vi "Colour selector.vi"(4 "Colour":string(combo), 11 "Error in":errorcluster) -> (15 "Error out":errorcluster)   [LabVIEW 2020]
uses:
  <vilib>/Utility/miscctls.llb/LVPositionTypeDef.ctl
panel:
  in  "Next":bool
  # "Catch and select the colour"
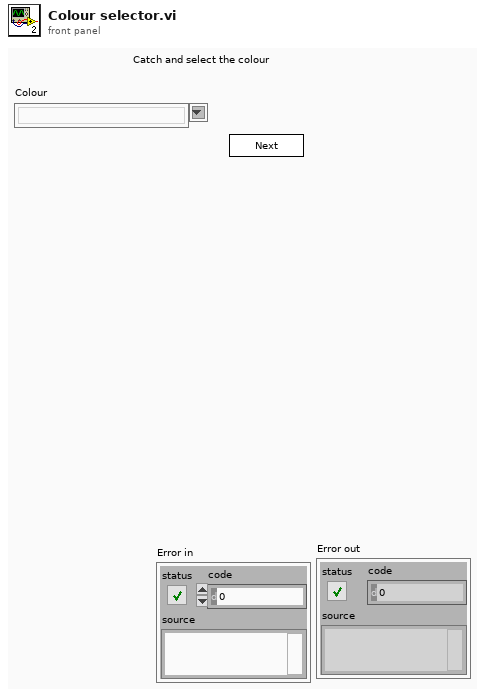
[diagram p1: front panel]
types:
  T1 = typedef "LVPositionTypeDef.ctl" = cluster{"Left":i32, "Top":i32}
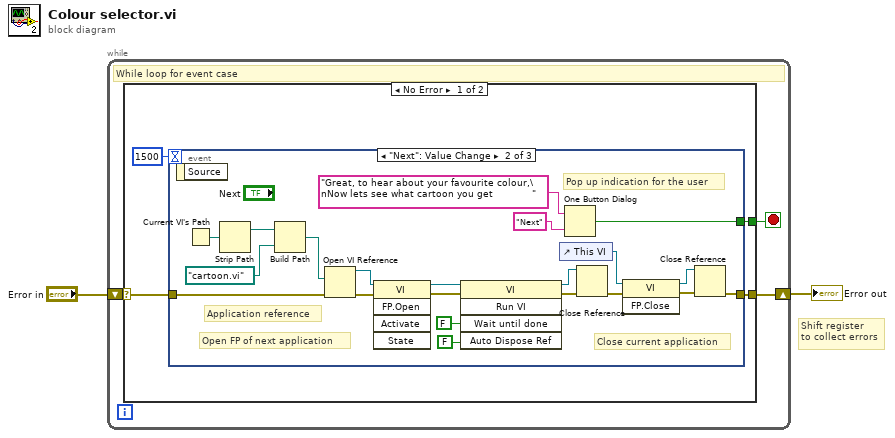
[diagram p0: block diagram]
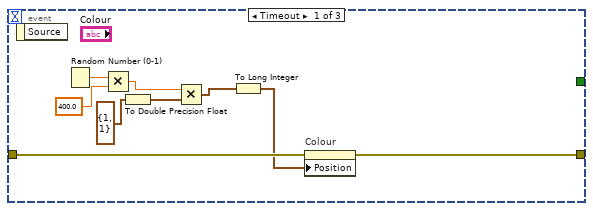
[diagram p2: hidden frame]
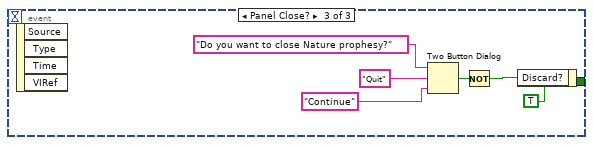
[diagram p3: hidden frame]
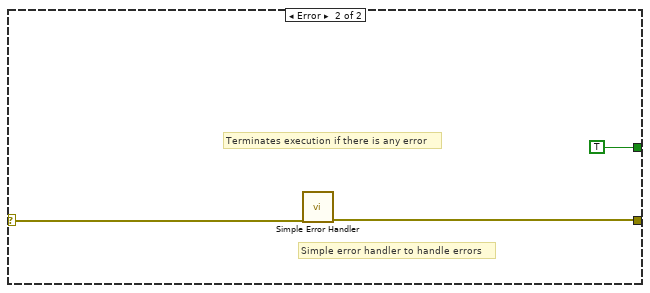
[diagram p4: hidden frame]
diagram:
  # "Shift register \nto collect errors"
  n1 = while {
    shift-right: [w4] -> w1
    shift-left: "Error in" -> [w5]
    stop <- w3 stop-if-true
    # "While loop for event case"
    n2 = case shown="No Error" w5 {
      selector: w5 -> [w9 w48]
      tunnel: [w8 w47] -> w4
      tunnel: [w7 TRUE] -> w3
      frame No Error {
        n3 = event shown="[1] \"Next\": Value Change" {
          selector: _ -> [_ _ _]
          dyn-events: _ -> [_ _ _]
          timeout: 1500 -> [_ _ _]
          tunnel: [w17 w26 _] -> w8
          tunnel: w9 -> [w18 w31 _]
          tunnel: [_ w25 TRUE] -> w7
          event Timeout {
            n4 = event-data() -> ()  [unwired: 1 in, 1 out]
            n5 = Random Number (0-1)() -> (number: 0 to 1=w16:dbl)
            n6 = Multiply(x=w16, y=400.0) -> (x*y=w14:dbl)
            n7 = To Double Precision Float(number=T1 {"Left"=1, "Top"=1} ("Position")) -> (double precision float=w13:cluster{"Left":dbl, "Top":dbl})
            n8 = Multiply(x=w14, y=w13) -> (x*y=w11:cluster{"Left":dbl, "Top":dbl})
            n9 = To Long Integer(number=w11) -> (32bit integer=w10:cluster{"Left":i32, "Top":i32})
            n10 = property on="Colour" class="CmbBox"(error in=w18, "Position"=w10) -> (error out=w17:errorcluster)  [unwired: 1 in, 1 out]
          }
          event "Next": Value Change {
            # "Pop up indication for the user"
            # "Close current application"
            # "Application reference"
            # "Open FP of next application"
            n11 = event-data() -> ()  [unwired: 1 in, 1 out]
            n12 = Current VI's Path() -> (path=w36:path)
            n13 = Strip Path(path=w36) -> (stripped path=w35:path)  [unwired: 1 out]
            n14 = Build Path(base path=w35, name or relative path=path "cartoon.vi") -> (appended path=w34:path)
            n15 = Open VI Reference(vi path=w34, error in (no error)=w31) -> (vi reference=w33:refnum<vi>, error out=w32:errorcluster)  [unwired: 4 in]
            n16 = invoke class="VI" method="FP.Open"(reference=w33, error in=w32) -> (reference out=w29:refnum<vi>, error out=w30:errorcluster)  [unwired: 3 in, 3 out]
            n17 = invoke class="VI" method="Run VI"(reference=w29, error in=w30, "Wait until done"=FALSE ("Wait Until Done"), "Auto Dispose Ref"=FALSE ("Auto Dispose Reference")) -> (reference out=w19:refnum<vi>, error out=w21:errorcluster)  [unwired: 1 in, 3 out]
            n18 = control-ref of="This VI"() -> (w22:refnum<vi>)
            n19 = One Button Dialog(message="Great, to hear about your favourite colour,\nNow lets see what cartoon you get             ", button name ("OK")="Next" ("T button name (\"OK\")")) -> (true=w25:bool)
            n20 = Close Reference(reference=w19, error in (no error)=w21) -> (error out=w20:errorcluster)
            n21 = invoke class="VI" method="FP.Close"(reference=w22, error in=w20) -> (reference out=w23:refnum<vi>, error out=w24:errorcluster)  [unwired: 1 in, 1 out]
            n22 = Close Reference(reference=w23, error in (no error)=w24) -> (error out=w26:errorcluster)
          }
          event Panel Close? {
            n23 = event-data() -> ()  [unwired: 1 in, 4 out]
            n24 = Two Button Dialog(message="Do you want to close Nature prophesy?", 1:"Continue" ("F button name (\"Cancel\")"), 2:"Quit" ("T button name (\"OK\")")) -> (T button?=w45:bool)
            n25 = Not(x=w45) -> (.not. x?=w44:bool)
            n26 = event-data("Discard?"=w44) -> ()  [unwired: 1 in, 1 out]
          }
        }
      }
      frame Error {
        # "Simple error handler to handle errors"
        # "Terminates execution if there is any error"
        n27 = call <vilib>:"Simple Error Handler.vi"("error in (no error)"=w48) -> ("error out"=w47:errorcluster)  [unwired: 4 in, 4 out]
      }
    }
  }
  "Error out" <- w1
